vi "SRV_FORLoop_End.vi"(2 "SuperPro":T1) -> (4 "SuperPro":T1)   [LabVIEW 2009]
doc: "End the closest for loop"
uses:
  <userlib>/SuperPro/OpCodes/_SubVIs/SuperProControl.ctl
panel:
  # "This LabVIEW item is deprecated.\n\nIt is believed to be unused and will be removed in a future version of SRV."
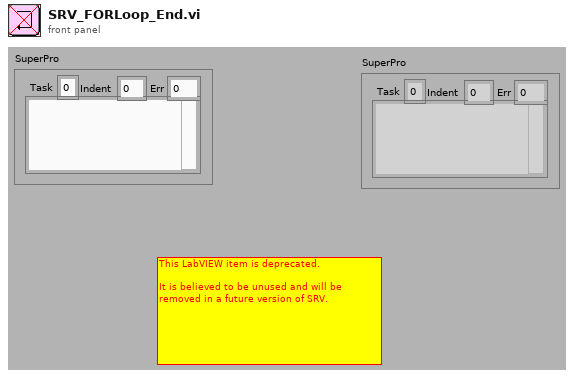
[diagram p1: front panel]
types:
  T1 = typedef "SuperProControl.ctl" = cluster{"Task":i32, "Indent":i32, "Err":i32, "ASM":string}
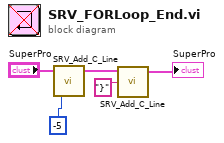
[diagram p0: block diagram]
diagram:
  n1 = call "SRV_Add_C_Line.vi"("inc"=-5 ("y"), "SuperPro in"="SuperPro") -> ("SuperPro out"=w1:T1)  [unwired: 3 in]
  n2 = call "SRV_Add_C_Line.vi"("C String"="}" ("format string"), "SuperPro in"=w1) -> ("SuperPro out"=→"SuperPro":T1)  [unwired: 3 in]
